vi "Restart Vision App.vi"(0 "adb location":string, 1 "error in":errorcluster) -> (2 "standard output":string, 3 "standard error":string, 4 "error out":errorcluster)   [LabVIEW 2016]
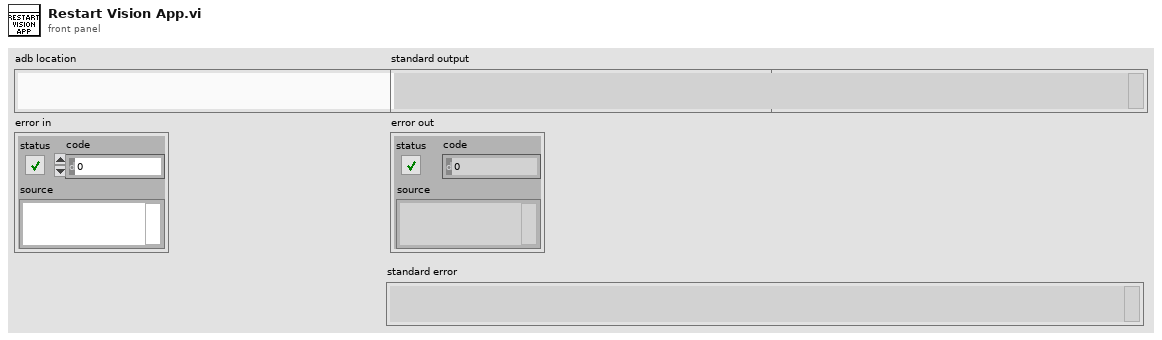
[diagram p1: front panel]
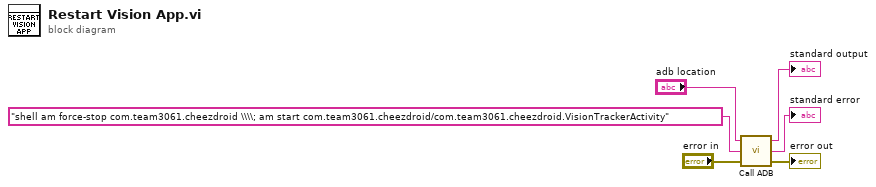
[diagram p0: block diagram]
diagram:
  n1 = call "Call ADB.vi"("error in"="error in", "adb sub-command"="shell am force-stop com.team3061.cheezdroid \\\\; am start com.team3061.cheezdroid/com.team3061.cheezdroid.VisionTrackerActivity", "adb location"="adb location") -> ("error out"=→"error out":errorcluster, "standard error"=→"standard error":string, "standard output"=→"standard output":string)
